vi "Lakeshore 218 Test Program.vi"() -> ()   [LabVIEW 2022 SP3]
uses:
  <instrlib>/Lake Shore Cryotronics 218/Lake Shore Cryotronics 218.lvlib
panel:
  out "error out":errorcluster
  out "Input Off/On":bool
  out "Input 1":dbl min=-9999.9 max=9999.9 step=0.0001 format="%.4f"
  in  "VISA resource name":refnum<visa-resource-name>="Lakeshore218"
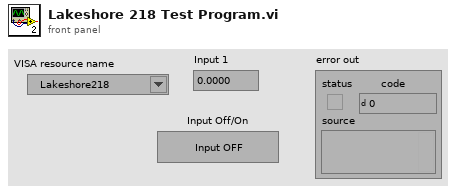
[diagram p1: front panel]
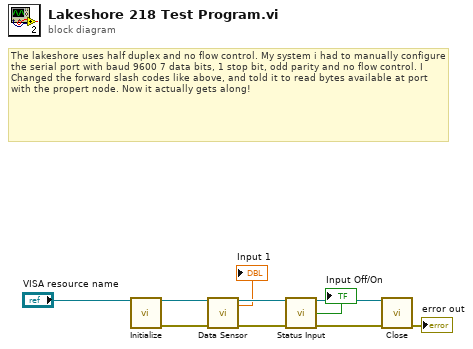
[diagram p0: block diagram]
diagram:
  # "The lakeshore uses half duplex and no flow control. My system i had to manually configure the serial port with baud 9600 7 data bits, 1 stop bit, odd parity and no flow control. I Changed the forward slash codes like above, and told it to read bytes available at port with the propert node. Now it actually gets along!"
  n1 = call <instrlib>:"Initialize.vi"("VISA resource name"="VISA resource name") -> ("VISA resource name out"=w6:refnum<visa-resource-name>, "error out"=w10:errorcluster)  [unwired: 13 in]
  n2 = call <instrlib>:"Data Sensor.vi"("VISA resource name"=w6, "error in (no error)"=w10) -> ("Input 1"=→"Input 1":dbl, "VISA resource name out"=w5:refnum<visa-resource-name>, "error out"=w9:errorcluster)  [unwired: 4 in, 7 out]
  n3 = call <instrlib>:"Status Input.vi"("VISA resource name"=w5, "error in (no error)"=w9) -> ("VISA resource name out"=w4:refnum<visa-resource-name>, "Input Off/On"=→"Input Off/On":bool, "error out"=w8:errorcluster)  [unwired: 9 in, 2 out]
  n4 = call <instrlib>:"Close.vi"("VISA resource name"=w4, "error in (no error)"=w8) -> ("error out"=→"error out":errorcluster)  [unwired: 13 in]
